vi "Obtain Strings.vi"(8 "error in":errorcluster, 11 "Custom Errors in":refnum<class "Custom Errors.lvclass">) -> (0 "error out":errorcluster, 1 "Strings":string[][](array[string]), 2 "Header":string[](array[string])=["Name", "Code", "Description"], 3 "Custom Errors out":refnum<class "Custom Errors.lvclass">)   [LabVIEW 2021, in "TAF Proj Document Type.lvlib" / "Custom Errors.lvclass"]
uses:
  <vilib>/Wovalab/AntiDoc/Document Type/Add-ons/LabVIEW TAF Project/Custom Errors/Custom Errors.lvclass
  <vilib>/Wovalab/AntiDoc/Document Type/Add-ons/LabVIEW TAF Project/Custom Errors/Custom Errors.lvclass/Custom Errors.ctl
  <vilib>/Wovalab/AntiDoc/Utilities/Utilities.lvlib
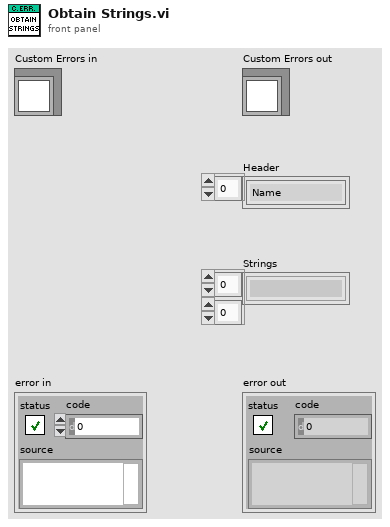
[diagram p1: front panel]
types:
  T1 = typedef "AntiDoc.lvlib/Bloc.lvclass/Custom Error Info--cluster.ctl" = cluster{"Code":i32, "Name":string, "Description":string, "Owned By":string[]}
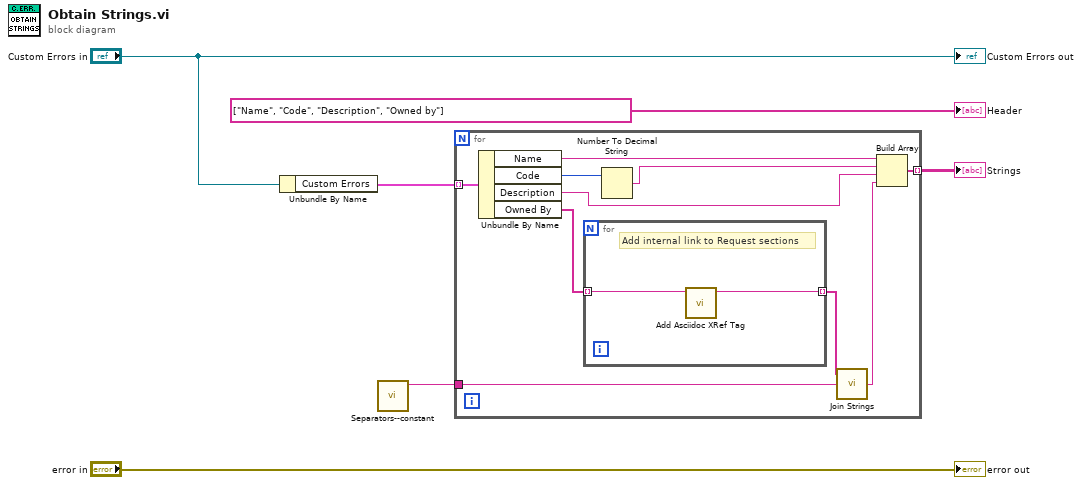
[diagram p0: block diagram]
diagram:
  n1 = Unbundle By Name("Custom Errors in") -> ("Custom Errors"=w4:T1[])
  n2 = call <vilib>:"Separators--constant.vi"() -> ("Caller Separator"=w1:string)  [unwired: 10 in, 1 out]
  n3 = for {
    tunnel: w4 -> [w16] mode=indexing
    tunnel: [w12] -> w3 mode=indexing
    tunnel: w1 -> [w9]
    n4 = Unbundle By Name(w16) -> ("Name"=w15:string, "Code"=w11:i32, "Description"=w13:string, "Owned By"=w8:string[])
    n5 = for {
      tunnel: w8 -> [w17] mode=indexing
      tunnel: [w18] -> w7 mode=indexing
      # "Add internal link to Request sections"
      n6 = call <vilib>:"Add Asciidoc XRef Tag.vi"("String In"=w17) -> ("String out"=w18:string)  [unwired: 10 in]
    }
    n7 = Number To Decimal String(number=w11) -> (decimal integer string=w14:string)  [unwired: 1 in]
    n8 = call <vilib>:"Join Strings.vi"("Separator (,)"=w9, "Strings In"=w7) -> ("String"=w10:string)  [unwired: 1 in]
    n9 = Build Array(w15, w14, w13, w10) -> (w12:string[])
  }
  "Strings" <- w3
  "error out" <- "error in"
  "Custom Errors out" <- "Custom Errors in"
  "Header" <- string[] ["Name", "Code", "Description", "Owned by"] ("Header")
